vi "Teleop.vi"(10 "Match Info":T1={"Autonomous Elapsed Seconds"=0.0, "TeleOp Elapsed Seconds"=0.0, "Disabled Elapsed Seconds"=0.0, "Visited Autonomous"=FALSE, "Visited TeleOp"=FALSE, "Visited Disabled"=FALSE, "Autonomous Settings"={"Autonomous Style"=enum."Independent", "VI Refnum"=refnum}}, 11 "Call Context":T2) -> ()   [LabVIEW 2013]
doc: "This VI is called for each TeleOp packet received from the DS where the robot is not disabled. It is often used to read from the joysticks and update I/O or to update setpoints for timed control loops. It should complete and return within 20 milliseconds or it may miss DS packets."
uses:
  <vilib>/Rock Robotics/WPI/DriverStation/WPI_DriverStationDerivedRobotMode.ctl
  <vilib>/Rock Robotics/WPI/DriverStation/WPI_DriverStationMatch Info.ctl
  Robot Global Data.vi
  <vilib>/Rock Robotics/WPI/RobotDrive/WPI_RobotDriveMecanumDrive_Cartesian.vi
  <vilib>/Rock Robotics/WPI/Joystick/WPI_JoystickGetSetRefNum.vi
  <vilib>/Rock Robotics/WPI/RobotDrive/WPI_RobotDriveGetSetRefNum.vi
panel:
  out "Numeric 1":dbl(slide) scale=0.0..100.0
  out "Boolean 2":bool
  out "Boolean 1":bool
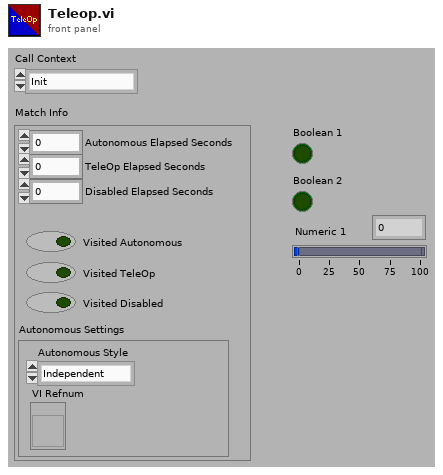
[diagram p1: front panel]
types:
  T1 = typedef "WPI_DriverStationMatch Info.ctl" = cluster{"Autonomous Elapsed Seconds":dbl, "TeleOp Elapsed Seconds":dbl, "Disabled Elapsed Seconds":dbl, "Visited Autonomous":bool, "Visited TeleOp":bool, "Visited Disabled":bool, "Autonomous Settings":cluster{"Autonomous Style":enum16{"Iterative", "Independent"}, "VI Refnum":refnum<vi>}}
  T2 = typedef "WPI_DriverStationDerivedRobotMode.ctl" = enum16{"Init", "Execute", "Stop"}
  T3 = typedef "WPI_RobotDriveDevRef.ctl" = cluster{"DevStatus":errorcluster, "Motors[]":T4[], "Square Inputs":bool, "Max Output":dbl, "Isochronous":bool}
  T4 = typedef "WPI_MotorControlDeviceRef.ctl" = cluster{"DeviceStatus":errorcluster, "Type":enum16{"PWM", "CAN"}, "PWM":cluster{"Digital Module":T5, "PWM Channel":T6, "DeadBand":T7}, "CAN":cluster{"Device Number":u8, "Control Mode":T8, "Semaphore":T9, "Max Vout":dbl}, "Invert":bool, "TransformRef":T10, "InvTransformRef":T10}
  T5 = typedef "FPGA_TypedefDigitalModule.ctl" = enum16{"Digital Module 1", "Digital Module 2"}
  T6 = typedef "FPGA_DIOPWMChannel.ctl" = enum8{"PWM 1", "PWM 2", "PWM 3", "PWM 4", "PWM 5", "PWM 6", "PWM 7", "PWM 8", "PWM 9", "PWM 10", "Invalid"}
  T7 = typedef "WPI_PWMDeadband.ctl" = cluster{"Name":string, "maxPositivePwm":i32, "minPositivePwm":i32, "centerPwm":i32, "maxNegativePwm":i32, "minNegativePwm":i32, "angularRange":u16}
  T8 = typedef "WPI_CANJaguar_ControlMode.ctl" = enum8{"Percent VBus", "Current", "Speed", "Position", "Voltage"}
  T9 = typedef "Semaphore RefNum" = refnum<k1>
  T10 = typedef "WPI_PWMTransform_ConPane.ctl" = refnum<vi>
  T11 = typedef "WPI_JoystickDevRef.ctl" = cluster{"Device":T12}
  T12 = typedef "WPI_JoystickDeviceEnum.ctl" = enum16{"USB 1", "USB 2", "USB 3", "USB 4", "Kinect 1", "Kinect 2"}
  T13 = typedef "WPI_JoystickButtonState.ctl" = cluster{"Button 1":bool, "Button 2":bool, "Button 3":bool, "Button 4":bool, "Button 5":bool, "Button 6":bool, "Button 7":bool, "Button 8":bool, "Button 9":bool, "Button 10":bool, "Button 11":bool, "Button 12":bool}
  T14 = cluster{"axis 1 (x)":dbl, "axis 2 (y)":dbl, "axis 3 (throttle)":dbl, "axis 4":dbl, "axis 5":dbl, "axis 6":dbl}
  T15 = typedef "WPI_ServoDeviceRef.ctl" = cluster{"DeviceStatus":errorcluster, "Digital Module":T5, "PWM Channel":T6, "DeadBand":T7}
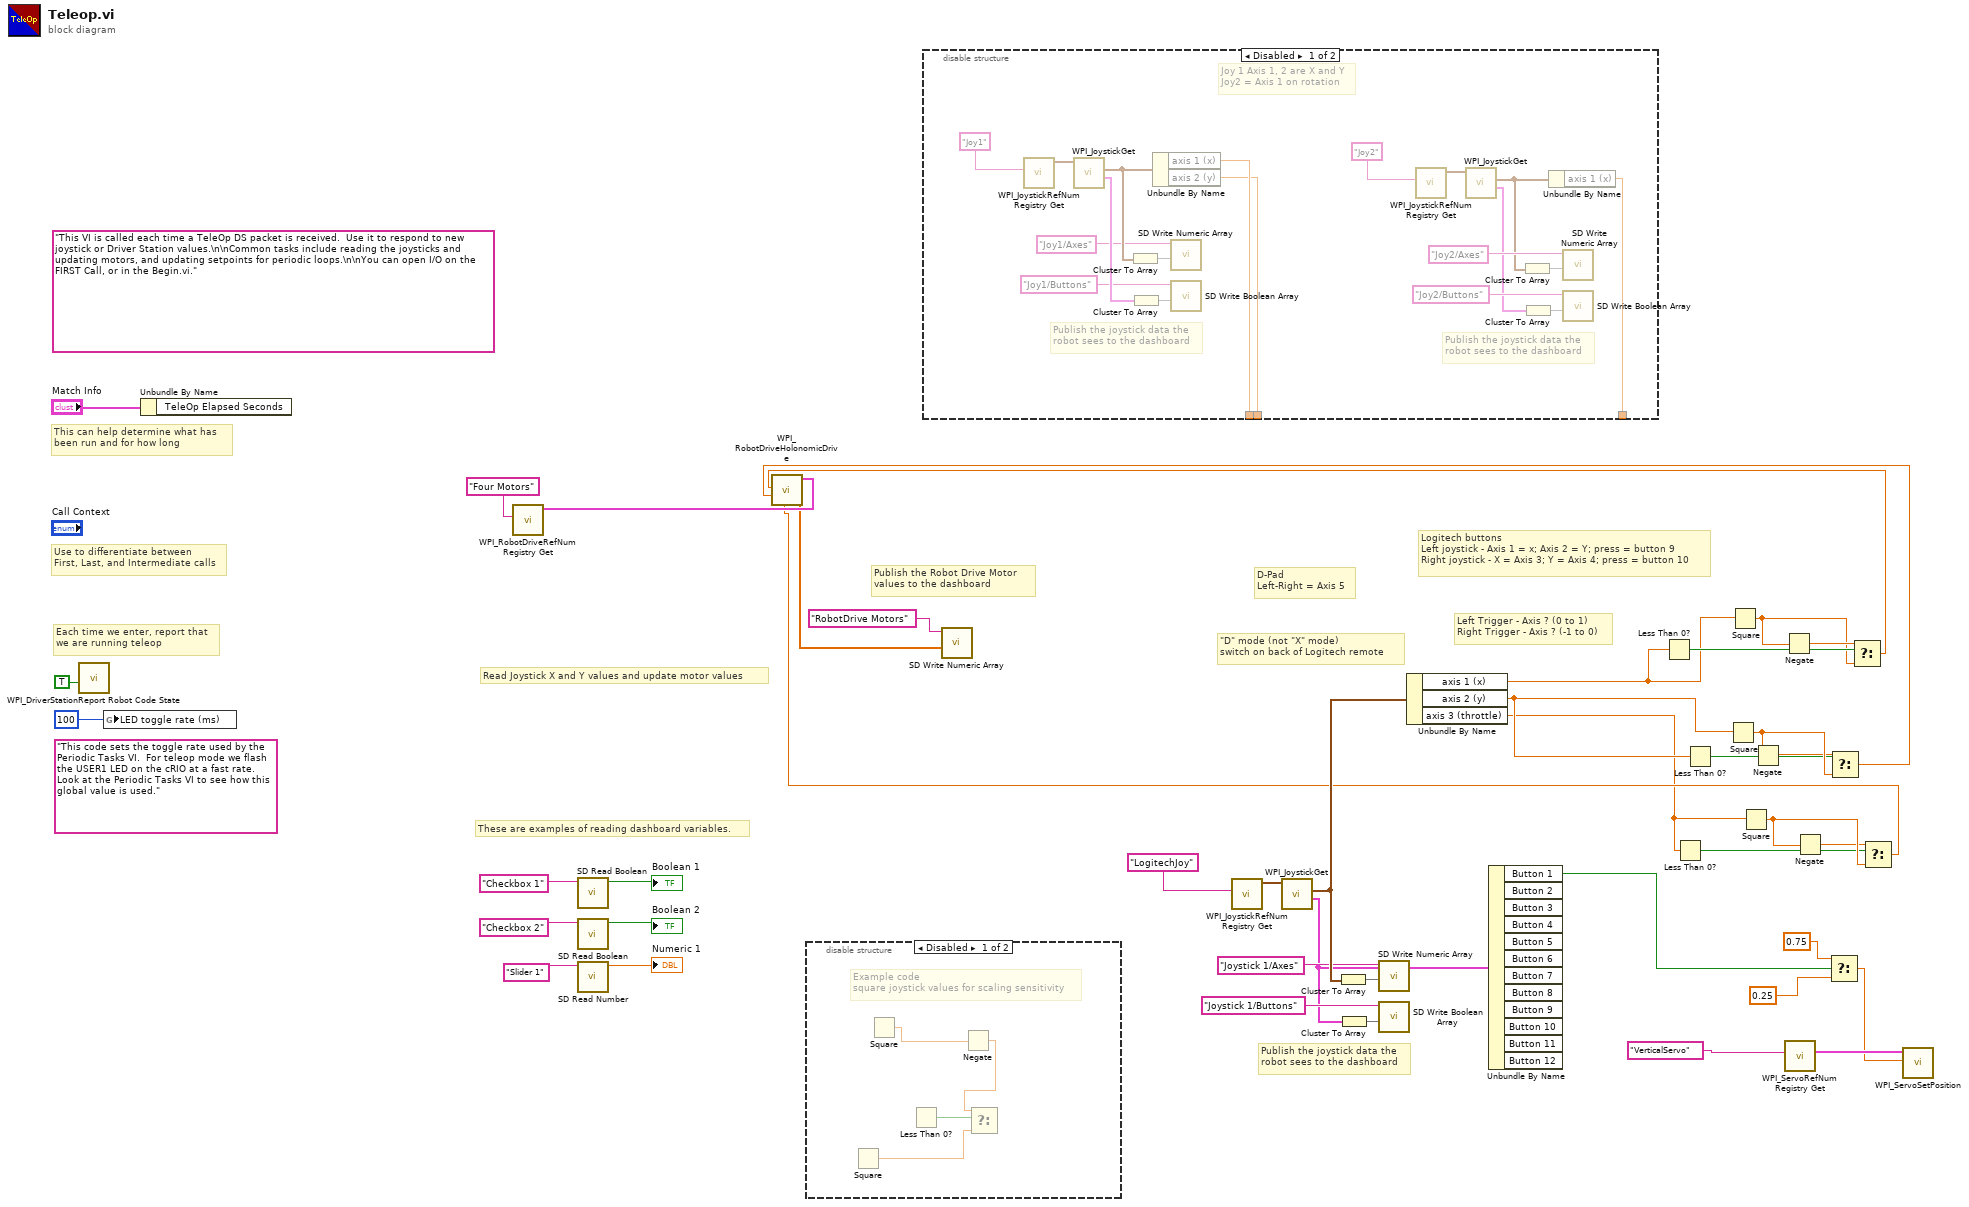
[diagram p0: block diagram]
diagram:
  (unwired) "This code sets the toggle rate used by the Periodic Tasks VI.  For teleop mode we flash the USER1 LED on the cRIO at a fast rate.  Look at the Periodic Tasks VI to see how this global value is used."
  (unwired) "This VI is called each time a TeleOp DS packet is received.  Use it to respond to new joystick or Driver Station values.\n\nCommon tasks include reading the joysticks and updating motors, and updating setpoints for periodic loops.\n\nYou can open I/O on the FIRST Call, or in the Begin.vi."
  # "\"D\" mode (not \"X\" mode)\nswitch on back of Logitech remote"
  # "D-Pad\nLeft-Right = Axis 5"
  # "Left Trigger - Axis ? (0 to 1)\nRight Trigger - Axis ? (-1 to 0)"
  # "Logitech buttons\nLeft joystick - Axis 1 = x; Axis 2 = Y; press = button 9\nRight joystick - X = Axis 3; Y = Axis 4; press = button 10"
  # "Publish the joystick data the\nrobot sees to the dashboard"
  # "These are examples of reading dashboard variables."
  # "Publish the Robot Drive Motor\nvalues to the dashboard"
  # "Each time we enter, report that\nwe are running teleop"
  # "Use to differentiate between\nFirst, Last, and Intermediate calls"
  # "This can help determine what has\nbeen run and for how long"
  # "Read Joystick X and Y values and update motor values"
  n1 = call <vilib>:"WPI_DriverStationReport Robot Code State.vi"("TeleOp"=TRUE ("Autonomous")) -> ()  [unwired: 10 in, 1 out]
  n2 = global write "Robot Global Data.vi" "LED toggle rate (ms)"(u32 100 ("LED ms toggle rate")) -> ()
  n3 = Unbundle By Name("Match Info") -> ()  [unwired: 1 out]
  n4 = call <vilib>:"WPI_RobotDriveRefNum Registry Get.vi"("refnum name"="Four Motors") -> ("RobotDriveDevRef"=w40:T3)  [unwired: 1 in, 9 out]
  n5 = call <vilib>:"SD Read Boolean.vi"("Name"="Checkbox 1" ("refnum name")) -> ("Boolean"=→"Boolean 1":bool)  [unwired: 8 in, 2 out]
  n6 = call <vilib>:"SD Read Boolean.vi"("Name"="Checkbox 2" ("refnum name")) -> ("Boolean"=→"Boolean 2":bool)  [unwired: 8 in, 2 out]
  n7 = call <vilib>:"SD Read Number.vi"("Name"="Slider 1" ("refnum name")) -> ("Numeric"=→"Numeric 1":dbl)  [unwired: 8 in, 2 out]
  n8 = disable-structure shown="Disabled" {
    frame Disabled {
      # "Example code\nsquare joystick values for scaling sensitivity"
      n9 = Square() -> (x^2=w44:dbl)  [unwired: 1 in]
      n10 = Square() -> (x^2=w45:dbl)  [unwired: 1 in]
      n11 = Less Than 0?() -> (x < 0?=w43:bool)  [unwired: 1 in]
      n12 = Negate(x=w45) -> (-x=w46:dbl)
      n13 = Select(t=w46, s=w43, f=w44) -> ()  [unwired: 1 out]
    }
    frame Enabled {
    }
  }
  n14 = disable-structure shown="Disabled" {
    disable-tunnel: [w65 _] -> _
    disable-tunnel: [w64 _] -> _
    disable-tunnel: [w48 _] -> _
    frame Disabled {
      # "Joy 1 Axis 1, 2 are X and Y\nJoy2 = Axis 1 on rotation"
      # "Publish the joystick data the\nrobot sees to the dashboard"
      # "Publish the joystick data the\nrobot sees to the dashboard"
      n15 = call <vilib>:"WPI_JoystickRefNum Registry Get.vi"("refnum name"="Joy1") -> ("JoystickDevRef"=w62:T11)  [unwired: 1 in, 9 out]
      n16 = call <vilib>:"WPI_JoystickGet.vi"("JoystickDevRef"=w62) -> ("Buttons"=w61:T13, "Axes"=w58:T14)  [unwired: 1 in, 4 out]
      n17 = Cluster To Array(cluster=w58) -> (array=w57:dbl[])
      n18 = Cluster To Array(cluster=w61) -> (array=w60:bool[])
      n19 = Unbundle By Name(w58) -> ("axis 1 (x)"=w65:dbl, "axis 2 (y)"=w64:dbl)
      n20 = call <vilib>:"SD Write Numeric Array.vi"("Numeric Array"=w57, "Name"="Joy1/Axes") -> ()  [unwired: 8 in, 2 out]
      n21 = call <vilib>:"SD Write Boolean Array.vi"("Boolean Array"=w60, "Name"="Joy1/Buttons") -> ()  [unwired: 8 in, 2 out]
      n22 = call <vilib>:"WPI_JoystickRefNum Registry Get.vi"("refnum name"="Joy2") -> ("JoystickDevRef"=w50:T11)  [unwired: 1 in, 9 out]
      n23 = call <vilib>:"WPI_JoystickGet.vi"("JoystickDevRef"=w50) -> ("Buttons"=w47:T13, "Axes"=w53:T14)  [unwired: 1 in, 4 out]
      n24 = Cluster To Array(cluster=w53) -> (array=w54:dbl[])
      n25 = Cluster To Array(cluster=w47) -> (array=w51:bool[])
      n26 = Unbundle By Name(w53) -> ("axis 1 (x)"=w48:dbl)
      n27 = call <vilib>:"SD Write Numeric Array.vi"("Numeric Array"=w54, "Name"="Joy2/Axes") -> ()  [unwired: 8 in, 2 out]
      n28 = call <vilib>:"SD Write Boolean Array.vi"("Boolean Array"=w51, "Name"="Joy2/Buttons") -> ()  [unwired: 8 in, 2 out]
    }
    frame Enabled {
    }
  }
  n29 = call <vilib>:"WPI_JoystickRefNum Registry Get.vi"("refnum name"="LogitechJoy") -> ("JoystickDevRef"=w28:T11)  [unwired: 1 in, 9 out]
  n30 = call <vilib>:"WPI_JoystickGet.vi"("JoystickDevRef"=w28) -> ("Buttons"=w22:T13, "Axes"=w25:T14)  [unwired: 1 in, 4 out]
  n31 = Cluster To Array(cluster=w25) -> (array=w24:dbl[])
  n32 = Cluster To Array(cluster=w22) -> (array=w27:bool[])
  n33 = call <vilib>:"SD Write Numeric Array.vi"("Numeric Array"=w24, "Name"="Joystick 1/Axes") -> ()  [unwired: 8 in, 2 out]
  n34 = call <vilib>:"SD Write Boolean Array.vi"("Boolean Array"=w27, "Name"="Joystick 1/Buttons") -> ()  [unwired: 8 in, 2 out]
  n35 = Unbundle By Name(w25) -> ("axis 1 (x)"=w18:dbl, "axis 2 (y)"=w14:dbl, "axis 3 (throttle)"=w7:dbl)
  n36 = Unbundle By Name(w22) -> ("Button 1"=w4:bool)  [unwired: 11 out]
  n37 = Less Than 0?(x=w18) -> (x < 0?=w21:bool)
  n38 = Less Than 0?(x=w7) -> (x < 0?=w11:bool)
  n39 = Less Than 0?(x=w14) -> (x < 0?=w15:bool)
  n40 = Square(x=w14) -> (x^2=w17:dbl)
  n41 = Square(x=w18) -> (x^2=w19:dbl)
  n42 = Square(x=w7) -> (x^2=w13:dbl)
  n43 = Negate(x=w17) -> (-x=w16:dbl)
  n44 = Negate(x=w19) -> (-x=w20:dbl)
  n45 = call <vilib>:"WPI_ServoRefNum Registry Get.vi"("refnum name"="VerticalServo") -> ("ServoDeviceRef"=w5:T15)  [unwired: 9 in, 1 out]
  n46 = Negate(x=w13) -> (-x=w12:dbl)
  n47 = Select(t=0.75, s=w4, f=0.25) -> (s? t:f=w1:dbl)
  n48 = Select(t=w16, s=w15, f=w17) -> (s? t:f=w8:dbl)
  n49 = Select(t=w20, s=w21, f=w19) -> (s? t:f=w9:dbl)
  n50 = Select(t=w12, s=w11, f=w13) -> (s? t:f=w10:dbl)
  n51 = call-poly <vilib>:"WPI_RobotDriveHolonomicDrive.vi"("Rotation"=w10, "Y"=w8, "X"=w9, "RobotDriveDevRef"=w40) -> ("Motor Values"=w36:dbl[])  [unwired: 5 in, 2 out]
  n52 = call <vilib>:"SD Write Numeric Array.vi"("Numeric Array"=w36, "Name"="RobotDrive Motors") -> ()  [unwired: 8 in, 2 out]
  n53 = call <vilib>:"WPI_ServoSetPosition.vi"("Position"=w1, "ServoDeviceRef"=w5) -> ()  [unwired: 8 in, 2 out]
